vi "BRig_Host_dataqueue__string__get.vi"(10 "input_errorDataQueue":errorcluster, 11 "input_hDataQueue":refnum<queue>) -> (0 "output_data":string, 1 "output_data":bool, 2 "output_errorDataQueue":errorcluster, 3 "output_hDataQueue":refnum<queue>)   [LabVIEW 2014]
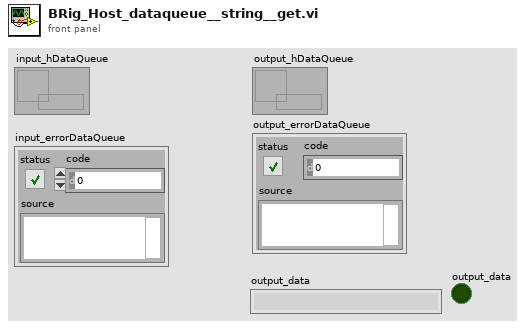
[diagram p1: front panel]
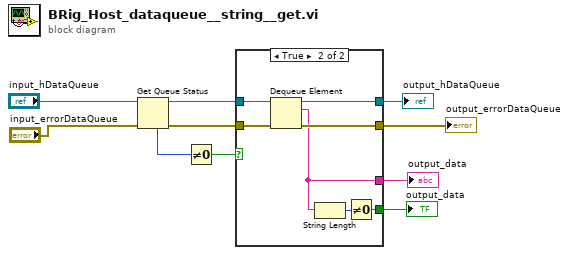
[diagram p0: block diagram]
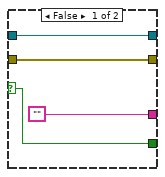
[diagram p2: hidden frame]
diagram:
  n1 = Get Queue Status(queue="input_hDataQueue", error in (no error)="input_errorDataQueue") -> (queue out=w6:refnum<queue>, error out=w5:errorcluster, # elements in queue=w8:i32)  [unwired: 1 in, 5 out]
  n2 = Not Equal To 0?(x=w8) -> (x != 0?=w7:bool)
  n3 = case shown="True" w7 {
    selector: w7 -> [w11 _]
    tunnel: w6 -> [w14 w21]
    tunnel: w5 -> [w13 w20]
    tunnel: [w14 w19] -> w4
    tunnel: [w13 w18] -> w3
    tunnel: ["" w17] -> w2
    tunnel: [w11 w15] -> w1
    frame False {
    }
    frame True {
      n4 = Dequeue Element(queue=w21, error in (no error)=w20) -> (queue out=w19:refnum<queue>, element=w17:string, error out=w18:errorcluster)  [unwired: 1 in, 1 out]
      n5 = String Length(string=w17) -> (length=w16:i32)
      n6 = Not Equal To 0?(x=w16) -> (x != 0?=w15:bool)
    }
  }
  "output_hDataQueue" <- w4
  "output_errorDataQueue" <- w3
  "output_data" <- w2
  "output_data" <- w1
